vi "Prepare Test Outputs.vi"(4 "Timing Metrics (\"\")":string, 5 "Save Results?":bool, 7 "Abort All":bool, 8 "error in (no error)":errorcluster, 9 "Message (\"\")":string, 10 "Status (\"\")":string, 11 "Results (\"\")":string) -> (3 "Test Output":T1)   [LabVIEW 2011]
uses:
  Test Output.ctl
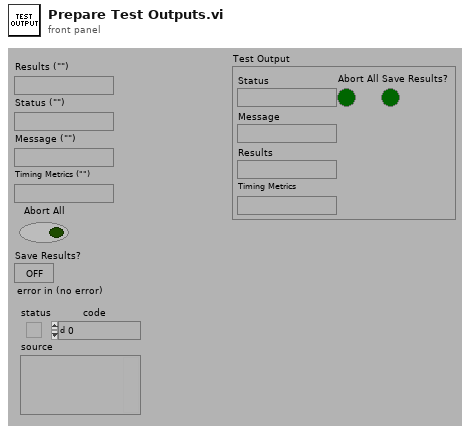
[diagram p1: front panel]
types:
  T1 = typedef "Test Output.ctl" = cluster{"Status":string, "Message":string, "Results":string, "Abort All":bool, "Save Results?":bool, "Timing Metrics":string}
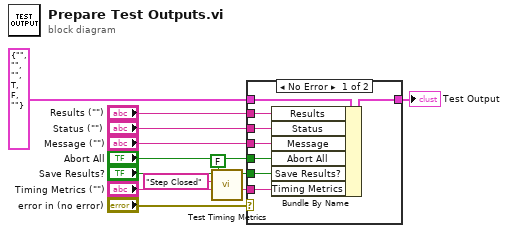
[diagram p0: block diagram]
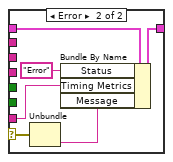
[diagram p2: hidden frame]
diagram:
  n1 = call "Test Timing Metrics.vi"("Start?"=FALSE, "Timing Metrics In"="Timing Metrics (\"\")", "Message"="Step Closed") -> ("Timing Metrics Out"=w1:string)  [unwired: 6 out]
  n2 = case shown="No Error" "error in (no error)" {
    selector: "error in (no error)" -> [_ w26]
    tunnel: "Results (\"\")" -> [w18 _]
    tunnel: "Status (\"\")" -> [w17 _]
    tunnel: "Message (\"\")" -> [w16 _]
    tunnel: T1 {"Status"="", "Message"="", "Results"="", "Abort All"=TRUE, "Save Results?"=FALSE, "Timing Metrics"=""} ("Test Output") -> [w20 w25]
    tunnel: [w19 w24] -> w7
    tunnel: "Abort All" -> [w15 _]
    tunnel: "Save Results?" -> [w14 _]
    tunnel: w1 -> [w13 w21]
    frame No Error {
      n3 = Bundle By Name(cluster=w20, "Results"=w18, "Status"=w17, "Message"=w16, "Abort All"=w15, "Save Results?"=w14, "Timing Metrics"=w13) -> (w19:T1)
    }
    frame Error {
      n4 = Unbundle(w26) -> ("source"=w22:string)  [unwired: 2 out]
      n5 = Bundle By Name(cluster=w25, "Status"="Error", "Timing Metrics"=w21, "Message"=w22) -> (w24:T1)
    }
  }
  "Test Output" <- w7
